vi "LoadSocketCommunication.vi"(0 "Universal Robot in":refnum<class "Universal Robot.lvclass">, 1 "Socket Communication":refnum<class "Socket Communication.lvclass">, 5 "error in (no error)":errorcluster) -> (14 "Universal Robot out":refnum<class "Universal Robot.lvclass">, 19 "error out":errorcluster)   [LabVIEW 2019, in "Universal Robot.lvclass"]
uses:
  Universal Robot.lvclass
  Client Interfaces/Socket Communication/Socket Communication.lvclass
  Universal Robot.lvclass/Universal Robot.ctl
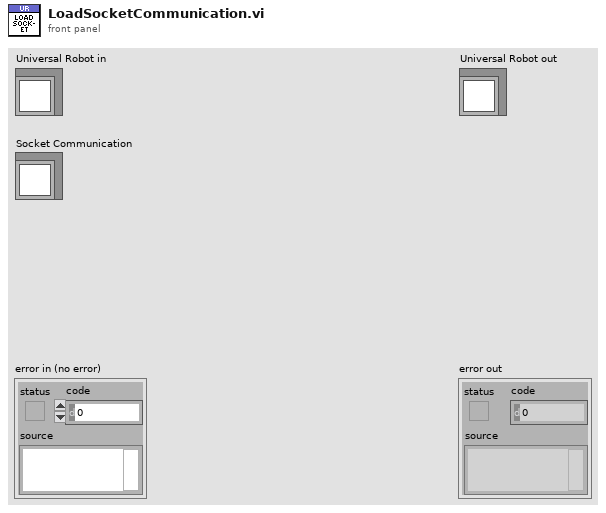
[diagram p1: front panel]
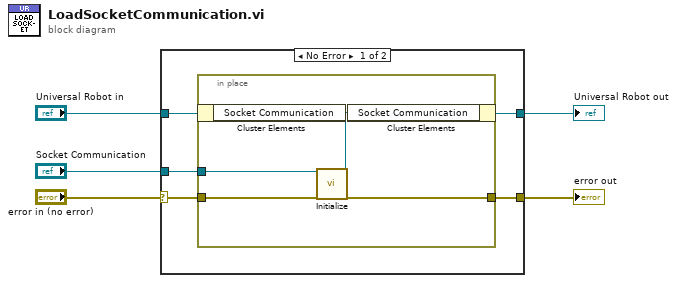
[diagram p0: block diagram]
diagram:
  n1 = case shown="No Error" "error in (no error)" {
    selector: "error in (no error)" -> [w10 w16]
    tunnel: [w9 w16] -> w4
    tunnel: [w7 w15] -> w2
    tunnel: "Universal Robot in" -> [w8 w15]
    tunnel: "Socket Communication" -> [w6 _]
    frame No Error {
      n2 = in-place {
        in-place-border: w10 -> [w14]
        in-place-border: [w11] -> w9
        in-place-border: w6 -> [w13]
        n3 = in-place-cluster #1(w8) -> ()  [unwired: 1 out]
        n4 = call-dynamic "Initialize.vi"("TCP Socket In"=w13, "error in (no error)"=w14) -> ("TCP Socket Out"=w12:refnum<class "Socket Communication.lvclass">, "error out"=w11:errorcluster)  [unwired: 16 in]
        n5 = in-place-cluster #1("Socket Communication"=w12) -> (w7:refnum<class "Universal Robot.lvclass">)
      }
    }
    frame Error {
    }
  }
  "error out" <- w4
  "Universal Robot out" <- w2
